vi "Math.Calculate, Vpp to Vrms.vi"(3 "Vpeak to peak":dbl) -> (0 "Vpeak":dbl, 1 "Vrms":dbl)   [LabVIEW 2024, in "EQMF.lvlib" / "Math Utils.lvlib"]
uses:
  Math Utils.lvlib
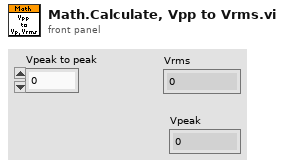
[diagram p1: front panel]
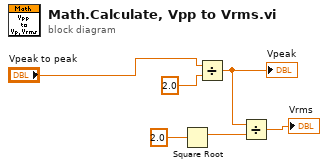
[diagram p0: block diagram]
diagram:
  n1 = Square Root(x=2.0) -> (sqrt(x)=w5:dbl)
  n2 = Divide(x="Vpeak to peak", y=2.0 ("x")) -> (x/y=w1:dbl)
  "Vpeak" <- w1
  n3 = Divide(x=w1, y=w5) -> (x/y=→"Vrms":dbl)
